vi "New Bomb.vi"(0 "Bomb in":refnum<class "Bomb.lvclass">[](array[class]), 1 "play sound":refnum<user-event>, 5 "Fruit":refnum<class "Fruit.lvclass">, 7 "Snake":refnum<class "Snake.lvclass">, 9 "B Game Size":u16, 11 "error in (no error)":errorcluster, 12 "Shield":refnum<class "Shield.lvclass">) -> (4 "Bomb out":refnum<class "Bomb.lvclass">[](array[class]), 6 "Position":cluster{"X":dbl, "Y":dbl}, 15 "error out":errorcluster)   [LabVIEW 2021, in "Bomb.lvclass"]
uses:
  Bomb.lvclass
  C:/Users/poche/Programs/LabVIEW/imposible snake/GameEl_class/GameEl.lvclass
  Snake_class/Snake.lvclass
  Fruit_class/Fruit.lvclass
  Shield/Shield.lvclass
  LVApp/Modules/Sound Manager/Typedefs/Sound Effects.ctl
  Snake_class/Snake.lvclass/Snake.ctl
  GameEl_class/GameEl.lvclass/GameEl.ctl
  GameEl_class/Read position.vi
  GameEl_class/Read Visible.vi
  Snake_class/Read Direction.vi
  Snake_class/Read Snake Head.vi
  GameEl_class/GameEl.lvclass
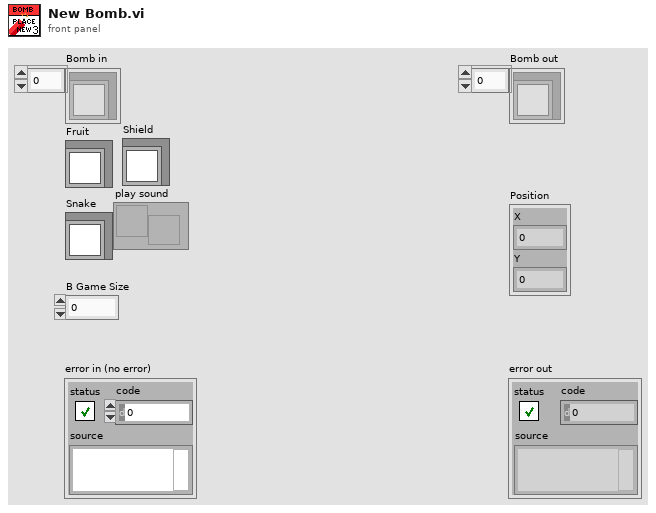
[diagram p1: front panel]
types:
  T1 = typedef "Sound Effects.ctl" = enum16{"Bomb In", "Bomb Out", "Bomb Touched", "Game Over", "Victory", "Eat", "10 Fruits", "Eat2", "Eat3", "Eat4", "MaxShield", "Shield", "10p", "Grape In", "Grape Out", "20p", "30p", "40p", "50p", "60p", "70p", "80p", "90p", "100p", "All shields cracked", "Mouse In", "Mouse Out", "Mouse Eaten", "Grape Eaten", "States Recover", "Broken Shield", "Bonus", "Happy Time", "explode", "Game over musica", "Back Music", "Shield Catch", "Evil lough", "Cricket In", "Cricket eaten", "Lets Go", "Jump1", "Jump2", "Jump3", "Unstoppable", "Troll Music", "winner"}
  T2 = typedef "GameEl.lvclass/Enum Direction.ctl" = enum16{"Up", "Down", "Forward", "Backward"}
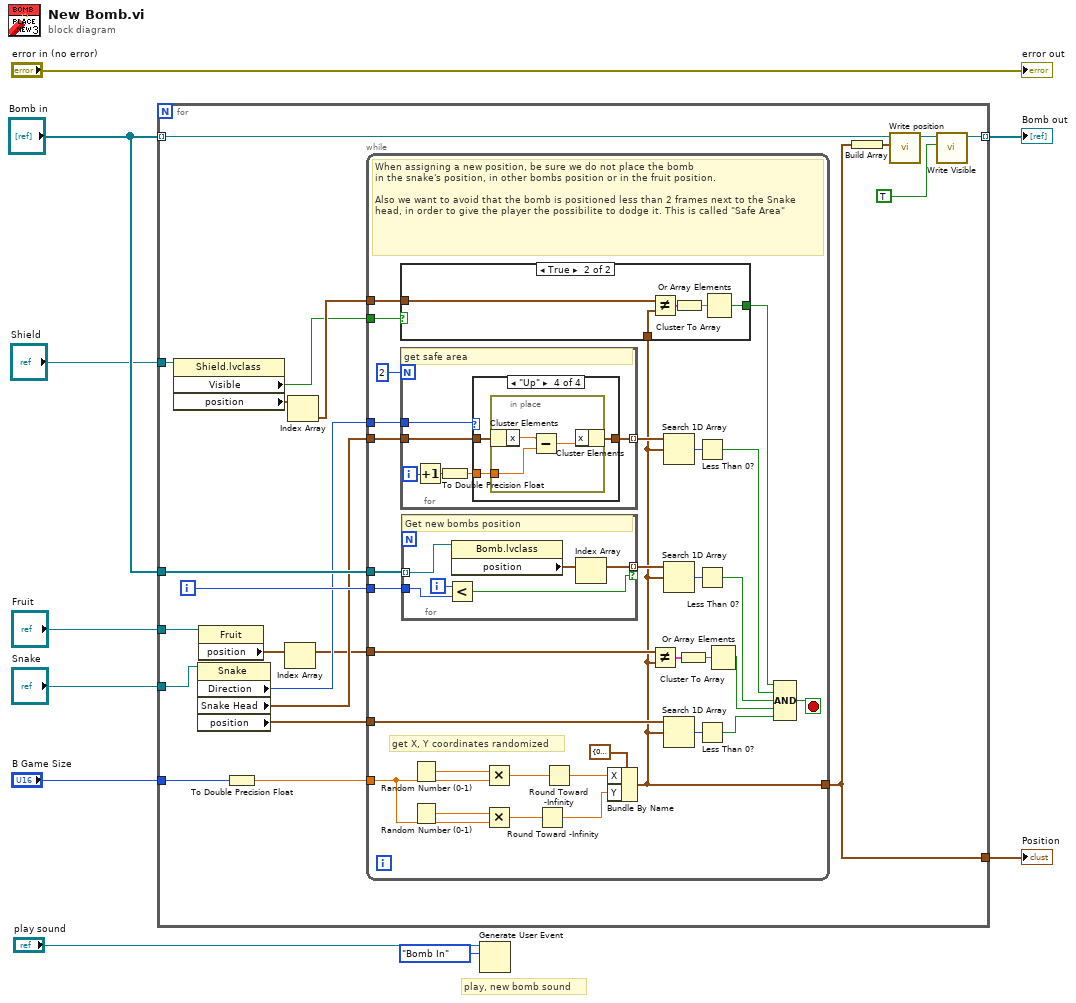
[diagram p0: block diagram]
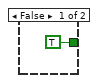
[diagram p2: hidden frame]
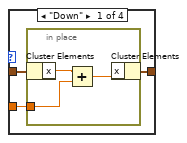
[diagram p3: hidden frame]
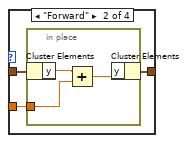
[diagram p4: hidden frame]
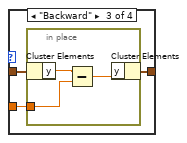
[diagram p5: hidden frame]
diagram:
  # "play, new bomb sound"
  n1 = for {
    tunnel: "B Game Size" -> [w31]
    tunnel: "Snake" -> [w25]
    tunnel: [w20] -> w8
    tunnel: "Bomb in" -> [w21] mode=indexing
    tunnel: [w16] -> w7 mode=indexing
    tunnel: "Fruit" -> [w28]
    tunnel: "Bomb in" -> [w27]
    tunnel: "Shield" -> [w14]
    i -> [w26]
    n2 = property class="Shield.lvclass"(reference=w14) -> ("Visible"=w11:bool, "position"=w13:cluster{"x":dbl, "y":dbl}[])  [unwired: 1 in, 2 out]
    n3 = property class="Snake"(reference=w25) -> ("Direction"=w24:T2, "Snake Head"=w22:cluster{"x":dbl, "y":dbl}, "position"=w23:cluster{"x":dbl, "y":dbl}[])  [unwired: 1 in, 2 out]
    n4 = property class="Fruit"(reference=w28) -> ("position"=w29:cluster{"x":dbl, "y":dbl}[])  [unwired: 1 in, 2 out]
    n5 = To Double Precision Float(number=w31) -> (double precision float=w30:dbl)
    n6 = Index Array(array=w29) -> (element=w15:cluster{"x":dbl, "y":dbl})  [unwired: 1 in]
    n7 = Index Array(array=w13) -> (element=w12:cluster{"x":dbl, "y":dbl})  [unwired: 1 in]
    n8 = while {
      tunnel: w30 -> [w60]
      tunnel: w23 -> [w53]
      tunnel: [w33] -> w20
      tunnel: w15 -> [w52]
      tunnel: w27 -> [w46]
      tunnel: w26 -> [w45]
      tunnel: w24 -> [w40]
      tunnel: w22 -> [w39]
      tunnel: w12 -> [w34]
      tunnel: w11 -> [w35]
      stop <- w49 stop-if-true
      # "get X, Y coordinates randomized"
      # "When assigning a new position, be sure we do not place the bomb \nin the snake's position, in other bombs position or in the fruit position.\n \nAlso we want to avoid that the bomb is positioned less than 2 frames next to the Snake head, in order to give the player the possibilite to dodge it. This is called \"Safe Area\""
      n9 = for {
        N: 2 -> [_]
        tunnel: w40 -> [w73]
        tunnel: w39 -> [w72]
        tunnel: [w69] -> w37 mode=indexing
        i -> [w74]
        # "get safe area"
        n10 = Increment(x=w74) -> (x+1=w71:i32)
        n11 = To Double Precision Float(number=w71) -> (double precision float=w70:dbl)
        n12 = case shown="\"Up\"" w73 {
          tunnel: w72 -> [w77 w83 w89 w95]
          tunnel: w70 -> [w76 w82 w88 w94]
          tunnel: [w75 w81 w87 w93] -> w69
          frame "Down" {
            n13 = in-place {
              in-place-border: w76 -> [w79]
              n14 = in-place-cluster #1(w77) -> ("x"=w80:dbl)
              n15 = Add(x=w80, y=w79) -> (x+y=w78:dbl)
              n16 = in-place-cluster #1("x"=w78) -> (w75:cluster{"x":dbl, "y":dbl})
            }
          }
          frame "Forward" {
            n17 = in-place {
              in-place-border: w82 -> [w85]
              n18 = in-place-cluster #2(w83) -> ("y"=w86:dbl)
              n19 = Add(x=w86, y=w85) -> (x+y=w84:dbl)
              n20 = in-place-cluster #2("y"=w84) -> (w81:cluster{"x":dbl, "y":dbl})
            }
          }
          frame "Backward" {
            n21 = in-place {
              in-place-border: w88 -> [w91]
              n22 = in-place-cluster #3(w89) -> ("y"=w92:dbl)
              n23 = Subtract(x=w92, y=w91) -> (x-y=w90:dbl)
              n24 = in-place-cluster #3("y"=w90) -> (w87:cluster{"x":dbl, "y":dbl})
            }
          }
          frame "Up" {
            n25 = in-place {
              in-place-border: w94 -> [w97]
              n26 = in-place-cluster #4(w95) -> ("x"=w98:dbl)
              n27 = Subtract(x=w98, y=w97) -> (x-y=w96:dbl)
              n28 = in-place-cluster #4("x"=w96) -> (w93:cluster{"x":dbl, "y":dbl})
            }
          }
        }
      }
      n29 = for {
        tunnel: w46 -> [w102] mode=indexing
        tunnel: w45 -> [w103]
        tunnel: [w99] -> w43 mode=indexing if=w100
        i -> [w104]
        # "Get new bombs position"
        n30 = Less?(x=w104, y=w103) -> (x < y?=w100:bool)
        n31 = property class="Bomb.lvclass"(reference=w102) -> ("position"=w101:cluster{"x":dbl, "y":dbl}[])  [unwired: 1 in, 2 out]
        n32 = Index Array(array=w101) -> (element=w99:cluster{"x":dbl, "y":dbl})  [unwired: 1 in]
      }
      n33 = Random Number (0-1)() -> (number: 0 to 1=w62:dbl)
      n34 = Random Number (0-1)() -> (number: 0 to 1=w61:dbl)
      n35 = Multiply(x=w62, y=w60) -> (x*y=w58:dbl)
      n36 = Multiply(x=w61, y=w60) -> (x*y=w57:dbl)
      n37 = Round Toward -Infinity(1:w57) -> (0:w54:dbl)
      n38 = Round Toward -Infinity(1:w58) -> (0:w55:dbl)
      n39 = Bundle By Name(cluster=cluster{"X":dbl, "Y":dbl} {"X"=0.0, "Y"=0.0} ("Position"), "X"=w55, "Y"=w54) -> (w33:cluster{"X":dbl, "Y":dbl})
      n40 = case shown="True" w35 {
        tunnel: w34 -> [_ w67]
        tunnel: w33 -> [_ w68]
        tunnel: [TRUE w64] -> w32
        frame False {
        }
        frame True {
          n41 = Not Equal?(x=w67, y=w68) -> (x != y?=w65:cluster{bool, bool})
          n42 = Cluster To Array(cluster=w65) -> (array=w66:bool[])
          n43 = Or Array Elements(Boolean array=w66) -> (logical OR=w64:bool)
        }
      }
      n44 = Not Equal?(x=w52, y=w33) -> (x != y?=w51:cluster{bool, bool})
      n45 = Search 1D Array(1D array=w37, element=w33) -> (index of element=w38:i32)  [unwired: 1 in]
      n46 = Search 1D Array(1D array=w43, element=w33) -> (index of element=w44:i32)  [unwired: 1 in]
      n47 = Search 1D Array(1D array=w53, element=w33) -> (index of element=w56:i32)  [unwired: 1 in]
      n48 = Cluster To Array(cluster=w51) -> (array=w50:bool[])
      n49 = Less Than 0?(x=w38) -> (x < 0?=w36:bool)
      n50 = Less Than 0?(x=w44) -> (x < 0?=w42:bool)
      n51 = Less Than 0?(x=w56) -> (x < 0?=w47:bool)
      n52 = Or Array Elements(Boolean array=w50) -> (logical OR=w48:bool)
      n53 = Compound Arithmetic op=AND(w32, w36, w42, w48, w47) -> (w49:bool)
    }
    n54 = Build Array(w20) -> (w19:cluster{"X":dbl, "Y":dbl}[])
    n55 = call "Write position.vi"("position"=w19, "GameEl in"=w21) -> ("GameEl out"=w18:refnum<class "Bomb.lvclass">)  [unwired: 8 in, 1 out]
    n56 = call "Write Visible.vi"("Visible"=TRUE, "GameEl in"=w18) -> ("GameEl out"=w16:refnum<class "Bomb.lvclass">)  [unwired: 8 in, 1 out]
  }
  "Bomb out" <- w7
  "Position" <- w8
  n57 = Generate User Event(user event="play sound", event data cluster=Sound_Effects."Bomb In" ("event data")) -> ()  [unwired: 2 in, 2 out]
  "error out" <- "error in (no error)"
